vi "CreateLogRecord.vi"(8 "error in (no error)":errorcluster, 9 "Message":string, 10 "Source":string, 11 "Level":T1(ring)=enum."Info") -> (0 "error out":errorcluster)   [LabVIEW 2016, in "Log4Lv.lvlib"]
doc: "Use this template to build a VI to use as a subVI."
uses:
  Log4Lv.lvlib
  Config Global.vi
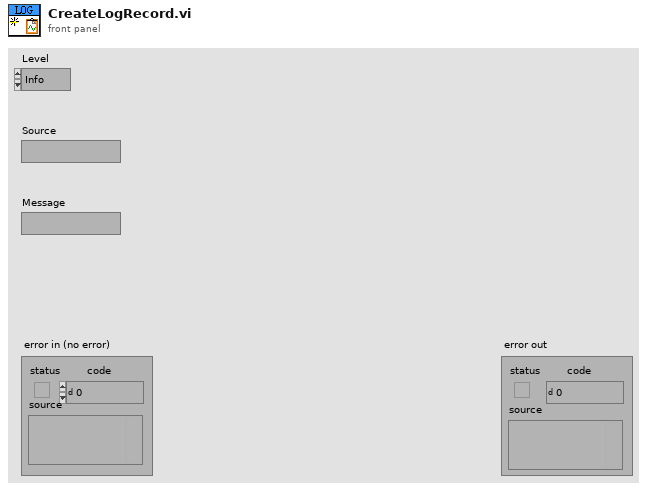
[diagram p1: front panel]
types:
  T1 = enum16{"Disable", "Error", "Warn", "Info", "Debug"}
  T2 = cluster{"LogName":string, "Level":enum16{"Disable", "Error", "Warn", "Info", "Debug"}, "LogFolder":path, "MaxFileSize":i32, "FileExtension":string, "TimeSytle":string, "LogStyle":string}
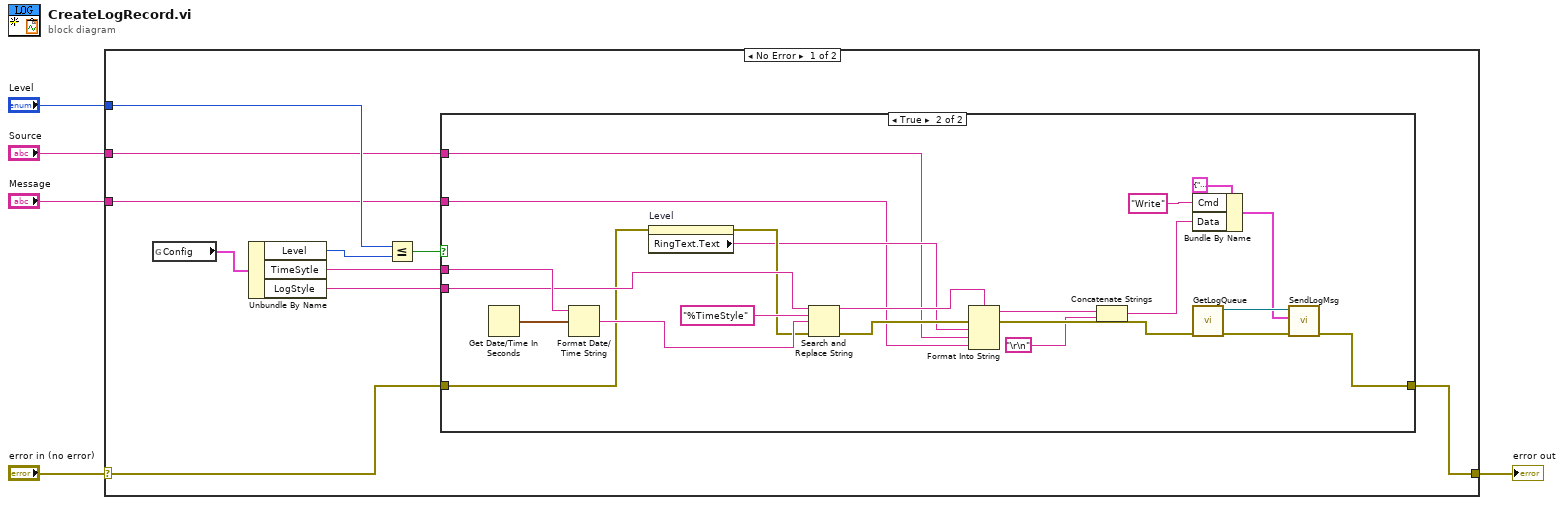
[diagram p0: block diagram]
diagram:
  n1 = case shown="No Error" "error in (no error)" {
    selector: "error in (no error)" -> [w7 w39]
    tunnel: [w6 w39] -> w4
    tunnel: "Level" -> [w14 _]
    tunnel: "Source" -> [w9 _]
    tunnel: "Message" -> [w8 _]
    frame No Error {
      n2 = global read "Config Global.vi" "Config"() -> (w15:T2)
      n3 = Unbundle By Name(w15) -> ("Level"=w13:T1, "TimeSytle"=w11:string, "LogStyle"=w10:string)
      n4 = Less Or Equal?(x=w14, y=w13) -> (x <= y?=w12:bool)
      n5 = case shown="True" w12 {
        tunnel: w11 -> [_ w37]
        tunnel: w10 -> [_ w34]
        tunnel: w9 -> [_ w18]
        tunnel: w8 -> [_ w17]
        tunnel: w7 -> [w16 w31]
        tunnel: [w16 w24] -> w6
        frame False {
        }
        frame True {
          n6 = Get Date/Time In Seconds() -> (seconds since 1Jan1904=w38:timestamp)
          n7 = Format Date/Time String(time format string (%c)=w37, seconds (now)=w38) -> (date/time string=w35:string)  [unwired: 1 in]
          n8 = property on="Level" class="Enum (strict)"(error in=w31) -> (error out=w33:errorcluster, "RingText.Text"=w19:string)  [unwired: 1 in, 1 out]
          n9 = Search and Replace String(input string=w34, search string="%TimeStyle", replace string=w35, error in=w33) -> (result string=w20:string, error out=w32:errorcluster)  [unwired: 4 in, 2 out]
          n10 = Format Into String(format string=w20, error in=w32, w19, w18, w17) -> (resulting string=w23:string, error out=w25:errorcluster)  [unwired: 1 in]
          n11 = Concatenate Strings(w23, "\r\n") -> (w21:string)
          n12 = Bundle By Name(cluster=cluster{"Cmd":string, "Data":variant} {"Cmd"="", "Data"=variant} ("LogMsg"), "Cmd"="Write", "Data"=w21) -> (w26:cluster{"Cmd":string, "Data":variant})
          n13 = call "GetLogQueue.vi"("error in (no error)"=w25) -> ("error out"=w30:errorcluster, "Queue Out"=w29:refnum<queue>)  [unwired: 9 in]
          n14 = call "SendLogMsg.vi"("error in (no error)"=w30, "LogMsg"=w26, "Queue In"=w29) -> ("error out"=w24:errorcluster)  [unwired: 7 in, 1 out]
        }
      }
    }
    frame Error {
    }
  }
  "error out" <- w4
